vi "Convert to Pascal Case.vi"(8 "error in (no error)":errorcluster, 11 "Input String":string) -> (0 "error out":errorcluster, 3 "Output String":string)   [LabVIEW 2015, in "Case Manipulation.lvlib"]
doc: "Introduction:\nWe often remove the spaces between words because programs of different sorts reserve the space (‘ ’) character for special purposes. Because the space character is reserved, we cannot use it to represent a concept that we express in our human language with multiple words.\nPascal Case:\nThis is also a very popular way to combine words to form a single concept. It is often used as a convention in declaring classes in many languages."
uses:
  Case Manipulation.lvlib
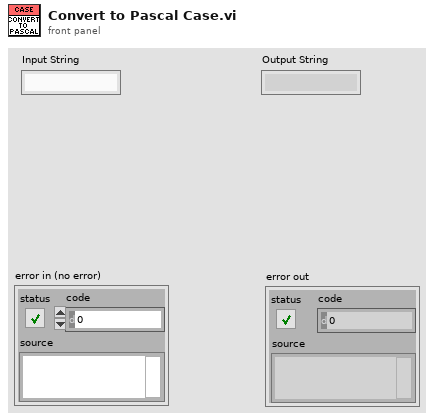
[diagram p1: front panel]
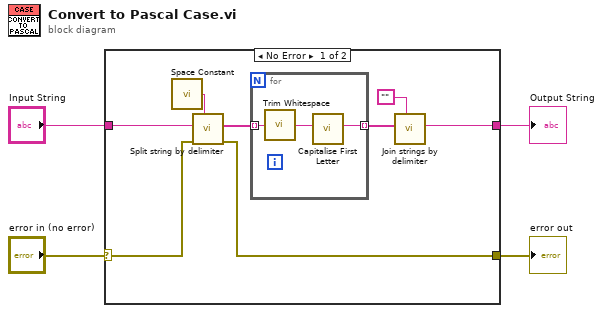
[diagram p0: block diagram]
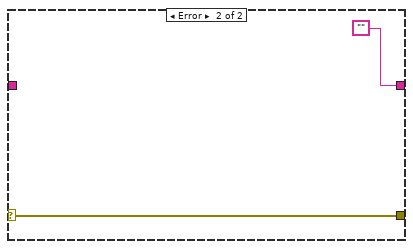
[diagram p2: hidden frame]
diagram:
  n1 = case shown="No Error" "error in (no error)" {
    selector: "error in (no error)" -> [w10 w16]
    tunnel: [w6 ""] -> w1
    tunnel: [w5 w16] -> w2
    tunnel: "Input String" -> [w12 _]
    frame No Error {
      n2 = call <vilib>:"Space Constant.vi"() -> ("String"=w11:string)
      n3 = call "Split string by delimiter.vi"("Delimiter"=w11, "error in (no error)"=w10, "String In"=w12) -> ("error out"=w5:errorcluster, "String Array Out"=w9:string[])  [unwired: 7 in]
      n4 = for {
        tunnel: w9 -> [w15] mode=indexing
        tunnel: [w14] -> w8 mode=indexing
        n5 = call <vilib>:"Trim Whitespace.vi"("string"=w15) -> ("trimmed string"=w13:string)  [unwired: 1 in]
        n6 = call "Capitalise First Letter.vi"("String In"=w13) -> ("String Out"=w14:string)  [unwired: 10 in]
      }
      n7 = call "Join strings by delimiter.vi"("Delimiter"="", "Strings []"=w8) -> ("String Out"=w6:string)  [unwired: 9 in]
    }
    frame Error {
    }
  }
  "error out" <- w2
  "Output String" <- w1
